vi "Read ChannelName.vi"(8 "error in (no error)":errorcluster, 11 "T560Channel in":refnum<class "T560Channel.lvclass">) -> (0 "error out":errorcluster, 2 "ChannelName":T1, 3 "T560Channel out":refnum<class "T560Channel.lvclass">)   [LabVIEW 2020, in "T560Channel.lvclass"]
uses:
  T560Channel.lvclass
  ChannelName.ctl
  T560Channel.lvclass/T560Channel.ctl
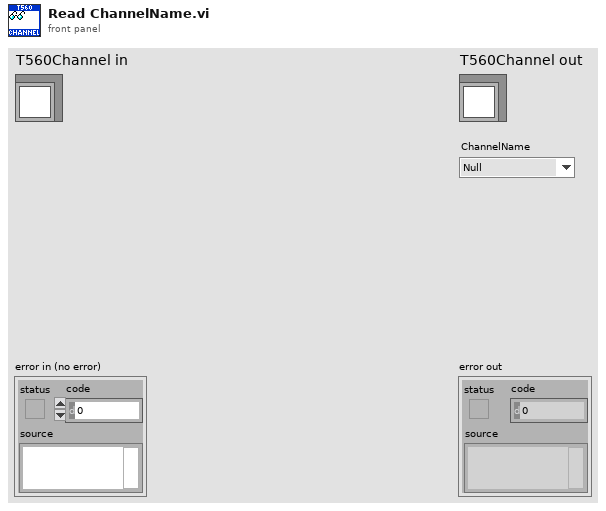
[diagram p1: front panel]
types:
  T1 = typedef "T560Channel.lvclass/ChannelName.ctl" = enum16{"Null", "A", "B", "C", "D", "Trigger"}
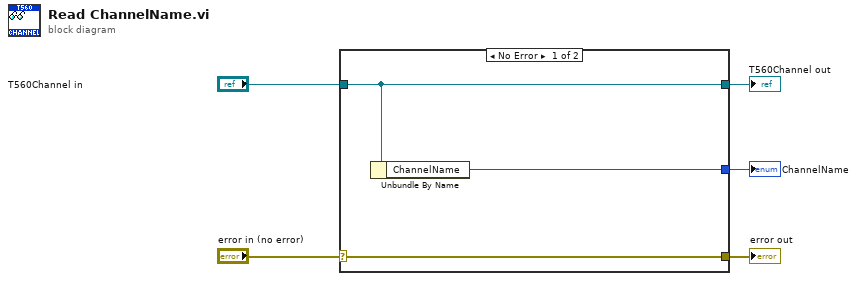
[diagram p0: block diagram]
diagram:
  n1 = case shown="No Error" "error in (no error)" {
    selector: "error in (no error)" -> [w8 w9]
    tunnel: [w8 w9] -> w4
    tunnel: [w7 w10] -> w2
    tunnel: "T560Channel in" -> [w7 w10]
    tunnel: [w6 _] -> w1
    frame No Error {
      n2 = Unbundle By Name(w7) -> ("ChannelName"=w6:T1)
    }
    frame Error {
    }
  }
  "error out" <- w4
  "T560Channel out" <- w2
  "ChannelName" <- w1
